vi "Next Step Selector.vi"(8 "error in":errorcluster, 11 "Car Wash Steps":string[][](array[string])) -> (0 "error out":errorcluster, 3 "Wash Steps Updated":string[][](array[string]), 5 "Step Status":string)   [LabVIEW 2020]
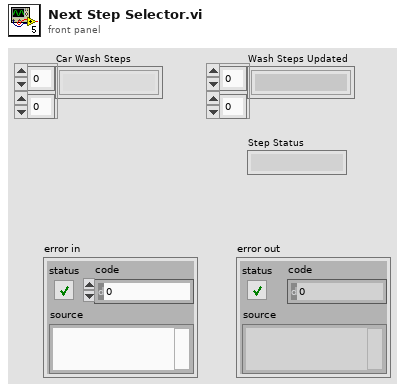
[diagram p1: front panel]
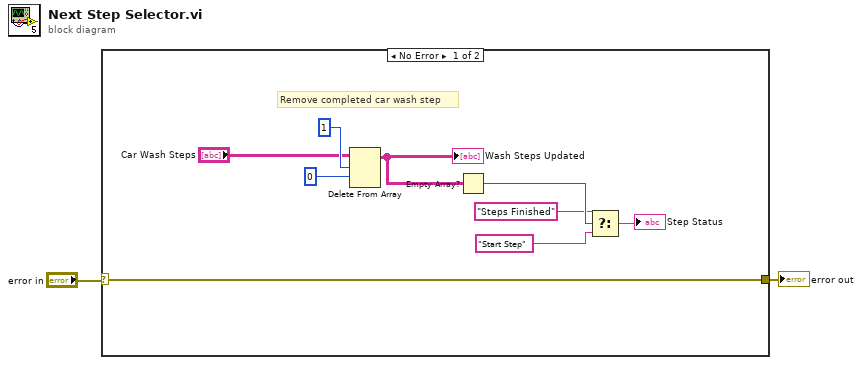
[diagram p0: block diagram]
diagram:
  n1 = case shown="No Error" "error in" {
    selector: "error in" -> [w6 w12]
    tunnel: [w6 w12] -> w1
    frame No Error {
      # "Remove completed car wash step"
      n2 = Delete From Array(array="Car Wash Steps", length=1, index (row)=0) -> (array with subset deleted=w10:string[][])  [unwired: 1 in, 1 out]
      "Wash Steps Updated" <- w10
      n3 = Empty Array?(array=w10) -> (empty?=w11:bool)
      n4 = Select(t="Steps Finished" ("New Step Status"), s=w11, f="Start Step" ("New Step Status")) -> (s? t:f=→"Step Status":string)
    }
    frame Error {
    }
  }
  "error out" <- w1
